vi "Relay_Read from FIFO.vi"(0 "FPGA VI Reference In":refnum<k20>, 1 "reset timestamp":bool, 5 "number of channels":u8, 7 "poll time [ms]":i32=10, 9 "system info in":refnum<class "EP System Info.lvclass">, 11 "error in (no error)":errorcluster) -> (4 "AI data":sgl[][](array[numeric]) format="%#.21g", 6 "sample rate [Hz]":sgl=9600.0 format="%#.6g", 8 "RT controler time":timestamp, 10 "system info out":refnum<class "EP System Info.lvclass">, 14 "elements remaining":u32, 15 "error out":errorcluster)   [LabVIEW 2016]
uses:
  <vilib>/addons/Electrical Power/PQ/Common/Classes/System Info/EP System Info.lvclass
  <vilib>/Analysis/baseanly.llb/Mean (DBL).vi
  <vilib>/Utility/error.llb/Error Cluster From Error Code.vi
  <vilib>/rvi/errors/niLvFpgaAdjustHostInterfaceError.vi
  <vilib>/rvi/interface/nirviMethod/nirviMethod.xnode
  <vilib>/FPGAPlugInAG/Dynamic/niLvFpga_ReadFifo_Dynamic.vi
  <vilib>/rvi/errors/niLvFpgaMergeErrorWithErrorCode.vi
  <vilib>/Analysis/NI_AALBase.lvlib
panel:
  in  "timeout (s)":dbl=5.0
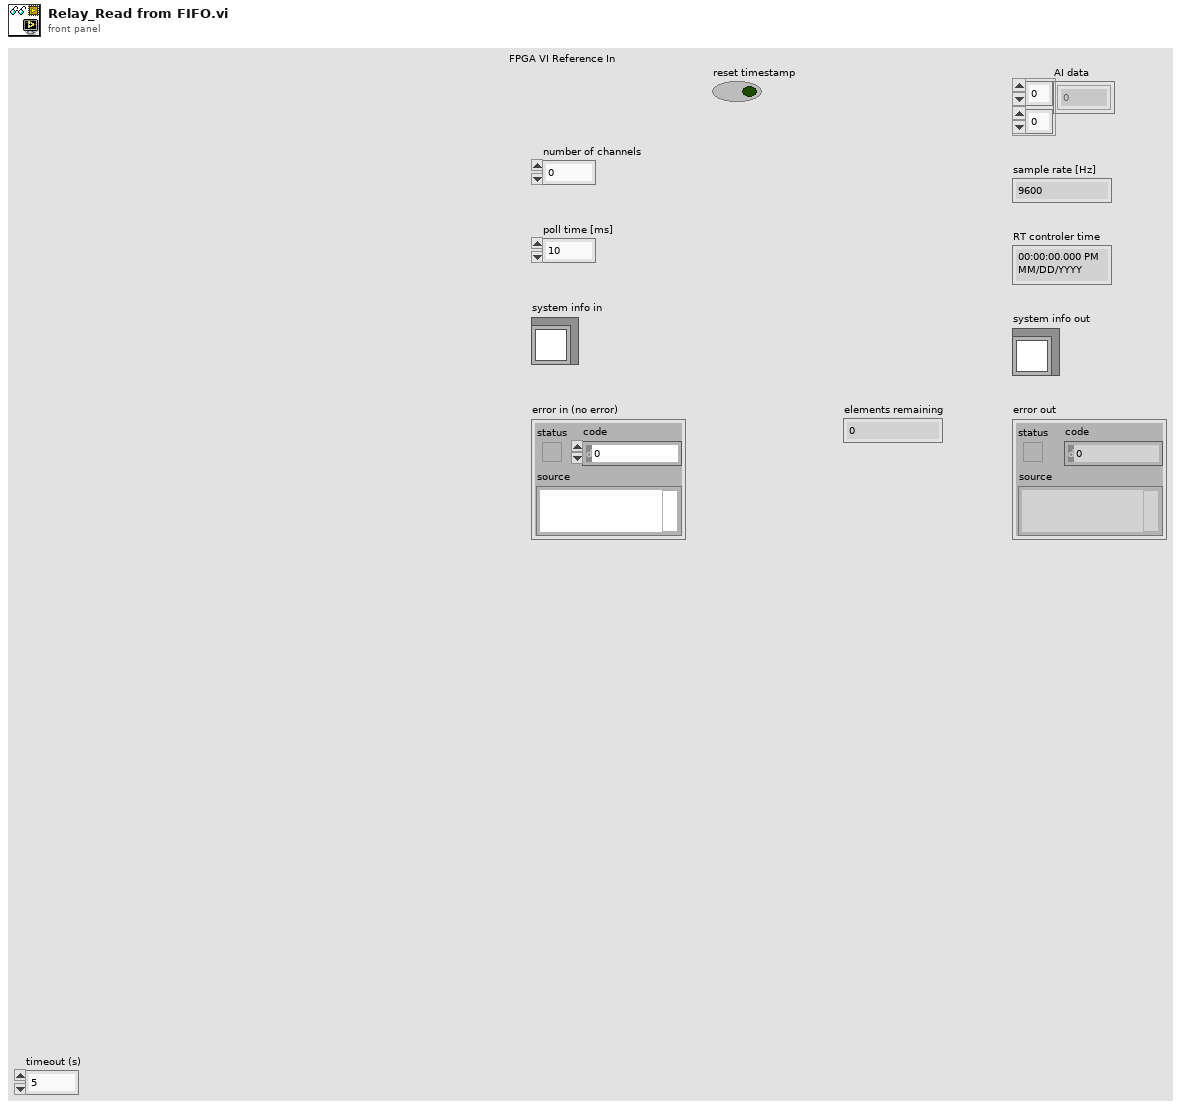
[diagram p1: front panel]
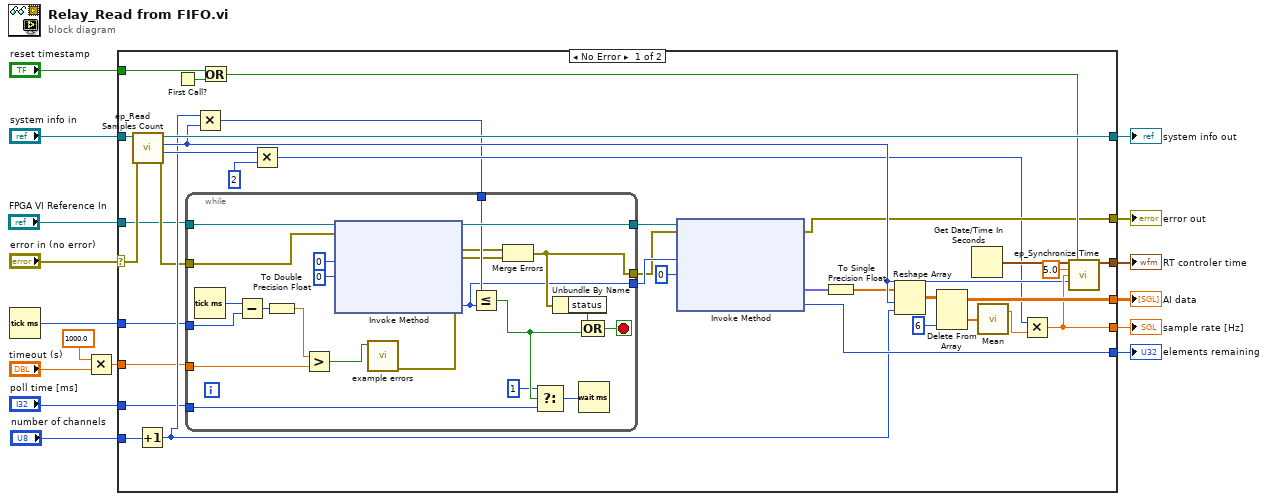
[diagram p0: block diagram]
diagram:
  n1 = Tick Count (ms)() -> (millisecond timer value=w5:u32)
  n2 = Multiply(x=1000.0 ("y"), y="timeout (s)") -> (x*y=w4:dbl)
  n3 = case shown="No Error" "error in (no error)" {
    selector: "error in (no error)" -> [w39 w75]
    tunnel: [w51 _] -> w16
    tunnel: [w47 w74] -> w15
    tunnel: [w50 _] -> w14
    tunnel: [w30 w75] -> w13
    tunnel: "system info in" -> [w40 w74]
    tunnel: [w49 _] -> w11
    tunnel: [w48 _] -> w10
    tunnel: "FPGA VI Reference In" -> [w20 _]
    tunnel: "reset timestamp" -> [w34 _]
    tunnel: w5 -> [w17 _]
    tunnel: w4 -> [w18 _]
    tunnel: "number of channels" -> [w28 _]
    tunnel: "poll time [ms]" -> [w19 _]
    frame No Error {
      n4 = call <vilib>:"ep_Read Samples Count.vi"("error in (no error)"=w39, "system info in"=w40) -> ("error out"=w23:errorcluster, "half-cycle (samples)"=w37:i32, "basic calc. interval (samples)"=w32:i32, "system info out"=w47:refnum<class "EP System Info.lvclass">)  [unwired: 5 in, 1 out]
      n5 = Increment(x=w28) -> (x+1=w27:u8)
      n6 = First Call?() -> (First Call?: T/F=w33:bool)
      n7 = Multiply(x=w27, y=w32) -> (x*y=w24:i32)
      n8 = while {
        tunnel: w17 -> [w71]
        tunnel: w18 -> [w68]
        tunnel: w23 -> [w66]
        tunnel: [w53] -> w22
        tunnel: [w62] -> w21
        tunnel: w20 -> [w63]
        tunnel: w24 -> [w61]
        tunnel: w19 -> [w57]
        tunnel: [w52] -> w25
        stop <- w64 stop-if-true
        n9 = Tick Count (ms)() -> (millisecond timer value=w73:u32)
        n10 = Subtract(x=w73, y=w71) -> (x-y=w72:u32)
        n11 = To Double Precision Float(number=w72) -> (double precision float=w69:dbl)
        n12 = Greater?(x=w69, y=w68) -> (0:w56:bool)
        n13 = xnode "Invoke Method"("FPGA VI Reference In"=w63, "error in"=w66, "Number of Elements"=u32 0, "Timeout (ms)"=0) -> ("FPGA VI Reference Out"=w62:refnum<k20>, "error out"=w55:errorcluster, "Elements Remaining"=w52:u32)  [unwired: 1 out]
        n14 = call <vilib>:"example errors.vi"("timeout?"=w56) -> ("error out"=w54:errorcluster)  [unwired: 10 in]
        n15 = Less Or Equal?(x=w61, y=w52) -> (x <= y?=w59:bool)
        n16 = Merge Errors(w55, w54) -> (w53:errorcluster)
        n17 = Select(t=1 ("index (row)"), s=w59, f=w57) -> (s? t:f=w60:i32)
        n18 = Unbundle By Name(w53) -> ("status"=w65:bool)
        n19 = Wait (ms)(milliseconds to wait=w60) -> ()  [unwired: 1 out]
        n20 = Compound Arithmetic op=OR(w65, w59) -> (w64:bool)
      }
      n21 = Or(x=w34, y=w33) -> (x .or. y?=w35:bool)
      n22 = Multiply(x=w37, y=2) -> (x*y=w26:i32)
      n23 = xnode "Invoke Method"("FPGA VI Reference In"=w21, "error in"=w22, "Number of Elements"=w25, "Timeout (ms)"=0) -> ("error out"=w30:errorcluster, "Data"=w46:fxp<+/-,26,5>[], "Elements Remaining"=w51:u32)  [unwired: 1 out]
      n24 = To Single Precision Float(number=w46) -> (single precision float=w29:sgl[])
      n25 = Reshape Array(w29, w32, w27) -> (w43:sgl[][])
      n26 = Delete From Array(array=w43, index (col)=6 ("index (row)")) -> (deleted portion=w45:sgl[], array with subset deleted=w50:sgl[][])  [unwired: 2 in]
      n27 = Get Date/Time In Seconds() -> (seconds since 1Jan1904=w44:timestamp)
      n28 = call-poly <vilib>:"Mean.vi"("X"=w45) -> ("mean"=w31:dbl)  [unwired: 1 out]
      n29 = Multiply(x=w26, y=w31) -> (x*y=w48:sgl)
      n30 = call <vilib>:"ep_Synchronize Time.vi"("RT controler time in"=w44, "reset"=w35, "maximum time difference (sec)"=5.0, "sampling rate (Hz)"=w48, "basic calc. interval (samples)"=w32) -> ("RT controler time out"=w49:timestamp)  [unwired: 10 in]
    }
    frame Error {
    }
  }
  "elements remaining" <- w16
  "system info out" <- w15
  "RT controler time" <- w11
  "sample rate [Hz]" <- w10
  "AI data" <- w14
  "error out" <- w13
